vi "Save Data.vi"(8 "error in (no error)":errorcluster, 10 "Data":T2, 11 "client handle in":T1) -> (0 "error out":errorcluster, 2 "Entry Id":string, 3 "client handle out":T1)   [LabVIEW 2019]
uses:
  <vilib>/httpClient/ClientHandle.ctl
  control/Solvestrive Store Data.ctl
  <vilib>/httpClient/POSTBuffer.vi
  <vilib>/httpClient/LabVIEWHTTPClient.lvlib
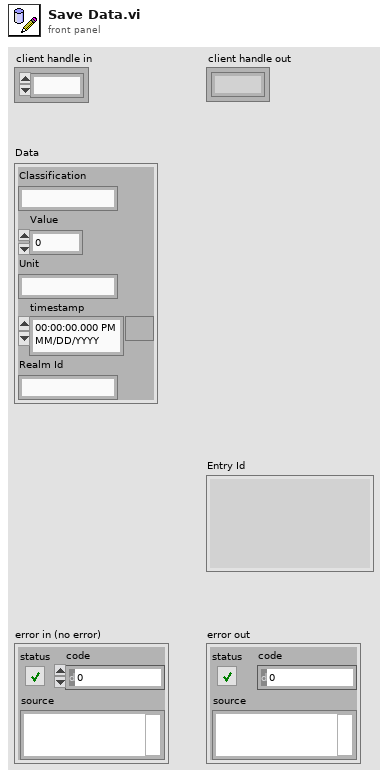
[diagram p1: front panel]
types:
  T1 = typedef "LabVIEWHTTPClient.lvlib/ClientHandle.ctl" = refnum<k1>
  T2 = typedef "Solvestrive Store Data.ctl" = cluster{"Classification":string, "Value":dbl, "Unit":string, "timestamp":timestamp, "Realm Id":string}
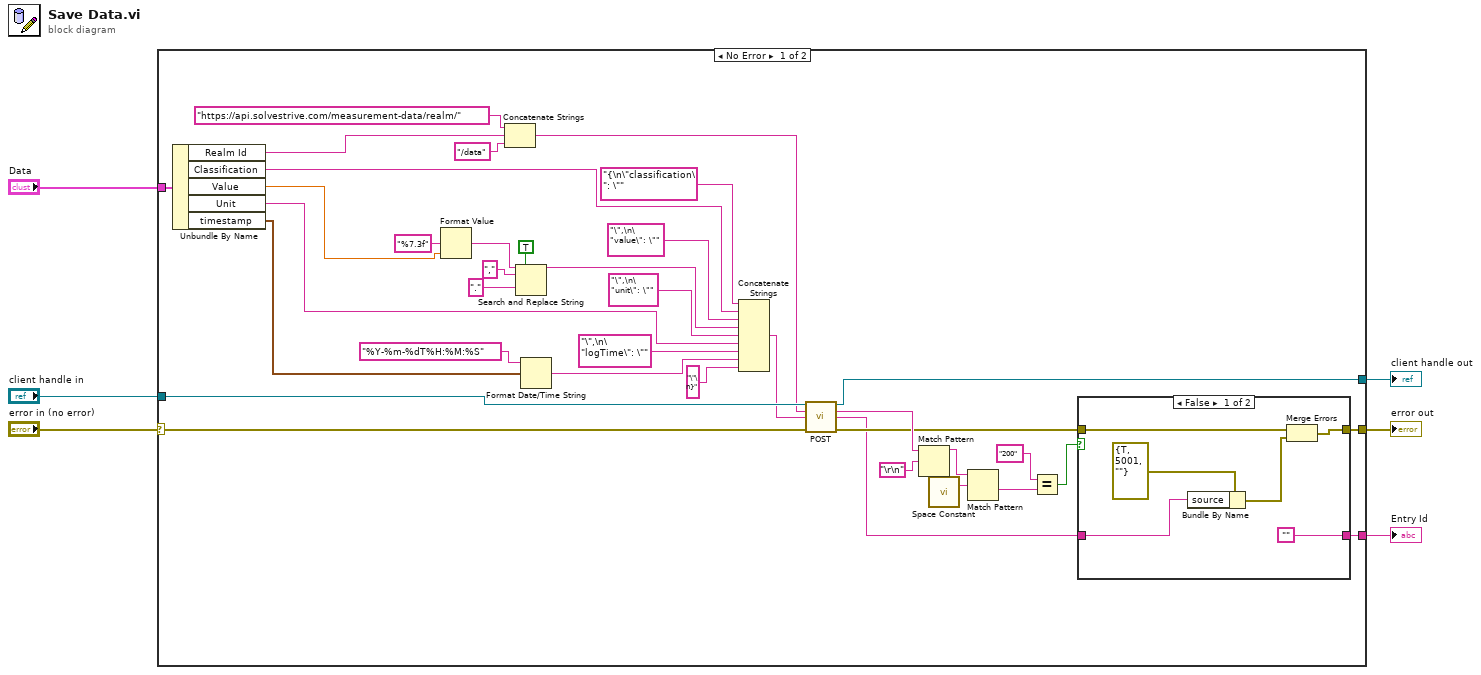
[diagram p0: block diagram]
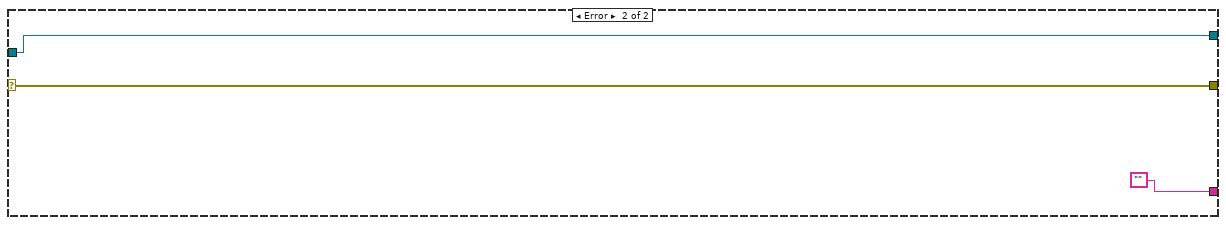
[diagram p3: hidden frame]
diagram:
  n1 = case shown="No Error" "error in (no error)" {
    selector: "error in (no error)" -> [w7 w54]
    tunnel: "client handle in" -> [w43 w53]
    tunnel: "Data" -> [w42 _]
    tunnel: [w19 w53] -> w4
    tunnel: [w12 w54] -> w3
    tunnel: [w8 ""] -> w2
    frame No Error {
      n2 = Unbundle By Name(w42) -> ("Realm Id"=w39:string, "Classification"=w36:string, "Value"=w29:dbl, "Unit"=w34:string, "timestamp"=w28:timestamp)
      n3 = Format Value(format string="%7.3f", value (0)=w29) -> (output string=w22:string)  [unwired: 1 in]
      n4 = Concatenate Strings("https://api.solvestrive.com/measurement-data/realm/" ("url"), w39, "/data" ("string")) -> (w41:string)
      n5 = Search and Replace String(replace all?=TRUE ("replace all? (F)"), input string=w22, search string=",", replace string="." ("replace string (\"\")")) -> (result string=w21:string)  [unwired: 4 in, 3 out]
      n6 = Format Date/Time String(time format string (%c)="%Y-%m-%dT%H:%M:%S", seconds (now)=w28) -> (date/time string=w27:string)  [unwired: 1 in]
      n7 = Concatenate Strings("{\n\"classification\": \"" ("buffer"), w36, "\",\n\"value\": \"" ("buffer"), w21, "\",\n\"unit\": \"" ("buffer"), w34, "\",\n\"logTime\": \"" ("buffer"), w27, "\"\n}" ("buffer")) -> (w20:string)
      n8 = call-poly <vilib>:"POST.vi"("client handle"=w43, "url"=w41, "buffer"=w20, "error in (no error)"=w7) -> ("client handle out"=w19:T1, "headers"=w18:string, "body"=w9:string, "error out"=w11:errorcluster)  [unwired: 8 in]
      n9 = Match Pattern(string=w18, regular expression="\r\n") -> (before substring=w17:string)  [unwired: 1 in, 3 out]
      n10 = call <vilib>:"Space Constant.vi"() -> ("String"=w16:string)
      n11 = Match Pattern(string=w17, regular expression=w16) -> (after substring=w14:string)  [unwired: 1 in, 3 out]
      n12 = Equal?(x="200", y=w14) -> (x = y?=w10:bool)
      n13 = case shown="False" w10 {
        tunnel: [w48 w51] -> w12
        tunnel: w11 -> [w47 w51]
        tunnel: w9 -> [w44 w50]
        tunnel: ["" w50] -> w8
        frame False {
          n14 = Bundle By Name(cluster=errorcluster {"status"=TRUE, "code"=5001, "source"=""} ("error constant"), "source"=w44) -> (w45:errorcluster)
          n15 = Merge Errors(w47, w45) -> (w48:errorcluster)
        }
        frame True {
        }
      }
    }
    frame Error {
    }
  }
  "Entry Id" <- w2
  "error out" <- w3
  "client handle out" <- w4
